vi "Initialize for Preview.vi"(8 "error in (no error)":errorcluster, 10 "Current Time":timestamp, 11 "Settings":T1={"Plug-in Version"="", "Step Values"=[], "Only Execute When Test Running"=TRUE, "Reset Sequence When Test Starts"=TRUE, "Number of Sequence Steps"=0, "Num of Analog Channels"=0, "Num of Digital Channels"=0, "Delay Before Starting Sequence"=0.0, "Default Analog Values"=[], "Default Digital Values"=[], "Max Iterations"=0, "Use last value when stopped"=FALSE, "Prioritize exact values"=FALSE, "Enable advanced step timing"=FALSE, "Enable step conditions"=FALSE, "Show confirmation dialogs"=FALSE, "Start condition"="", "Enable re-triggering"=FALSE, "Stop condition"=""}) -> (0 "error out":errorcluster, 3 "Output Sequencer out":refnum<class "Output Sequencer.lvclass">)   [LabVIEW 2020, in "Output Sequencer.lvlib" / "Output Sequencer.lvclass"]
uses:
  Output Sequencer.lvclass
  Settings UI/Types/Settings.ctl
  Settings UI/Types/Step Settings.ctl
  Types/Sequencer State.ctl
  Output Sequencer.lvclass/Output Sequencer.ctl
  Settings UI/Settings UI.lvclass
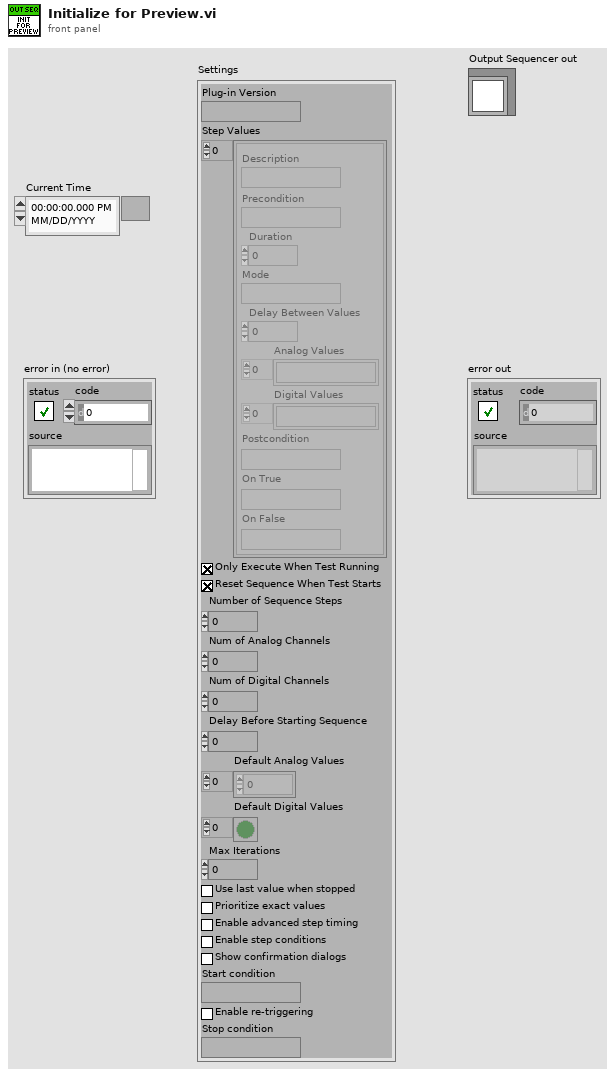
[diagram p1: front panel]
types:
  T1 = typedef "Output Sequencer.lvlib/Settings UI.lvclass/Settings.ctl" = cluster{"Plug-in Version":string, "Step Values":T2[], "Only Execute When Test Running":bool, "Reset Sequence When Test Starts":bool, "Number of Sequence Steps":i32, "Num of Analog Channels":i32, "Num of Digital Channels":i32, "Delay Before Starting Sequence":dbl, "Default Analog Values":dbl[], "Default Digital Values":bool[], "Max Iterations":u32, "Use last value when stopped":bool, "Prioritize exact values":bool, "Enable advanced step timing":bool, "Enable step conditions":bool, "Show confirmation dialogs":bool, "Start condition":string, "Enable re-triggering":bool, "Stop condition":string}
  T2 = typedef "Output Sequencer.lvlib/Settings UI.lvclass/Step Settings.ctl" = cluster{"Description":string, "Precondition":string, "Duration":dbl, "Mode":string, "Delay Between Values":dbl, "Analog Values":string[], "Digital Values":string[], "Postcondition":string, "On True":string, "On False":string}
  T3 = typedef "Output Sequencer.lvlib/Output Sequencer.lvclass/Sequencer State.ctl" = enum16{"Error", "Initialize", "Prepare channels", "Wait for test", "Wait for %.1f sec", "Wait for trigger", "Stop condition", "Wait for resume", "Running", "Paused", "No valid step", "Stopped"}
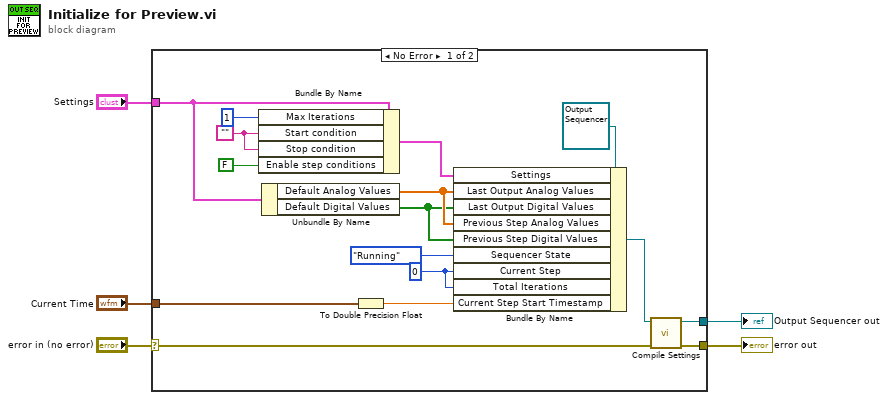
[diagram p0: block diagram]
diagram:
  n1 = case shown="No Error" "error in (no error)" {
    selector: "error in (no error)" -> [w9 w22]
    tunnel: [w8 w22] -> w4
    tunnel: [w6 _] -> w3
    tunnel: "Settings" -> [w10 _]
    tunnel: "Current Time" -> [w18 _]
    frame No Error {
      w13 = 0 ("Total Iterations")
      w16 = ""
      n2 = Bundle By Name(cluster=w10, "Max Iterations"=u32 1, "Start condition"=w16, "Stop condition"=w16, "Enable step conditions"=FALSE) -> (w11:T1)
      n3 = Unbundle By Name(w10) -> ("Default Analog Values"=w20:dbl[], "Default Digital Values"=w19:bool[])
      n4 = To Double Precision Float(number=w18) -> (double precision float=w12:dbl)
      n5 = Bundle By Name(cluster=refnum<class "Output Sequencer.lvclass"> refnum ("Sequencer with Output Values out"), "Settings"=w11, "Last Output Analog Values"=w20, "Last Output Digital Values"=w19, "Previous Step Analog Values"=w20, "Previous Step Digital Values"=w19, "Sequencer State"=Sequencer_State."Running" ("State.Sequencer State"), "Current Step"=w13, "Total Iterations"=w13, "Current Step Start Timestamp"=w12) -> (w7:refnum<class "Output Sequencer.lvclass">)
      n6 = call "Compile Settings.vi"("error in (no error)"=w9, "Plugin in"=w7) -> ("error out"=w8:errorcluster, "Plugin out"=w6:refnum<class "Output Sequencer.lvclass">)  [unwired: 8 in]
    }
    frame Error {
    }
  }
  "error out" <- w4
  "Output Sequencer out" <- w3
